vi "Set Margin.vi"(8 "error in (no error)":errorcluster, 9 "Margin":T1={"Type"=1, "Width"=40, "Sensitive"=TRUE, "Mask"=0, "Cursor"=2} {"Cursor" items=["Arrow"=2, "ReverseArrow"=7]; "Type" items=["Symbol", "Number", "BackColor", "ForeColor", "Text", "RightText", "Color"]}, 10 "Index":i32=1, 11 "ScintillaNET in":refnum<class "ScintillaNET.lvclass">) -> (0 "error out":errorcluster, 3 "ScintillaNET out":refnum<class "ScintillaNET.lvclass">)   [LabVIEW 2018, in "ScintillaNET.lvclass"]
uses:
  ScintillaNET.lvclass
  ScintillaNET.lvclass/ScintillaNET.ctl
  D:/project/hobby/LF2R/LabVIEW/source/ScintillaNET/dll/ScintillaNET.dll
  dll/ScintillaNET.dll
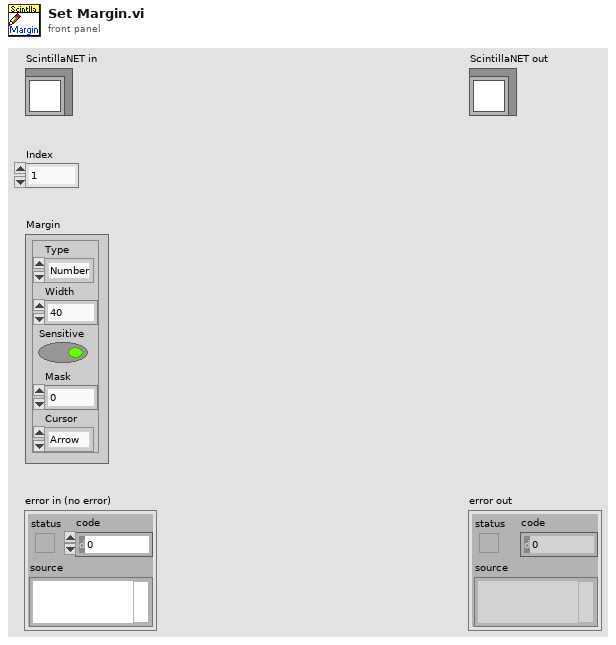
[diagram p1: front panel]
types:
  T1 = cluster{"Type":i32, "Width":i32, "Sensitive":bool, "Mask":u32, "Cursor":i32}
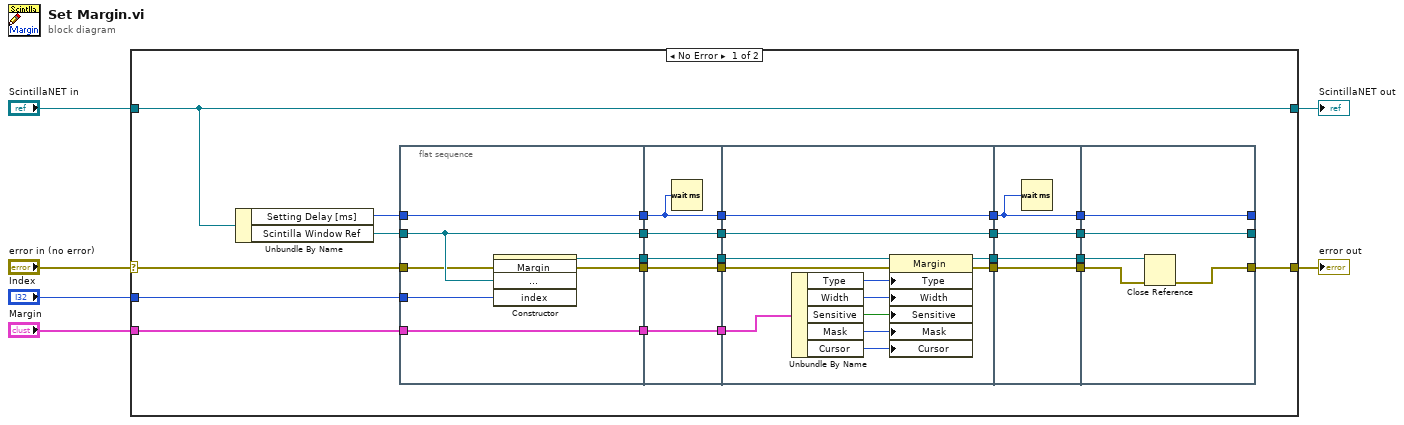
[diagram p0: block diagram]
diagram:
  n1 = case shown="No Error" "error in (no error)" {
    selector: "error in (no error)" -> [w8 w66]
    tunnel: [w7 w66] -> w5
    tunnel: [w15 w65] -> w3
    tunnel: "ScintillaNET in" -> [w15 w65]
    tunnel: "Margin" -> [w12 _]
    tunnel: "Index" -> [w11 _]
    frame No Error {
      n2 = Unbundle By Name(w15) -> ("Setting Delay [ms]"=w13:u32, "Scintilla Window Ref"=w14:refnum<k24>)
      n3 = flat-sequence {
        tunnel: w14 -> [w36]
        tunnel: [w38] -> w31
        tunnel: [w37] -> w30
        tunnel: [w36] -> w29
        tunnel: [w35] -> w28
        tunnel: w13 -> [w35]
        tunnel: w12 -> [w33]
        tunnel: w11 -> [w34]
        tunnel: [w33] -> w9
        tunnel: w8 -> [w32]
        tunnel: w31 -> [w43]
        tunnel: w30 -> [w42]
        tunnel: w29 -> [w41]
        tunnel: [w43] -> w27
        tunnel: [w42] -> w26
        tunnel: [w41] -> w25
        tunnel: w28 -> [w40]
        tunnel: [w40] -> w24
        tunnel: [w39] -> w10
        tunnel: w9 -> [w39]
        tunnel: w27 -> [w51]
        tunnel: w26 -> [w50]
        tunnel: w25 -> [w55]
        tunnel: w24 -> [w54]
        tunnel: [w52] -> w23
        tunnel: [w55] -> w22
        tunnel: [w54] -> w21
        tunnel: [w53] -> w20
        tunnel: w10 -> [w49]
        tunnel: w23 -> [w58]
        tunnel: w22 -> [w57]
        tunnel: w21 -> [w56]
        tunnel: w20 -> [w59]
        tunnel: [w59] -> w19
        tunnel: [w58] -> w18
        tunnel: [w57] -> w17
        tunnel: [w56] -> w16
        tunnel: [w63] -> _
        tunnel: [w64] -> _
        tunnel: w19 -> [w62]
        tunnel: w18 -> [w61]
        tunnel: w17 -> [w64]
        tunnel: w16 -> [w63]
        tunnel: [w60] -> w7
        frame #0 {
          n4 = constructor class="Margin"(error in=w32, "scintilla"=w36, "index"=w34) -> (reference out=w38:refnum<k24>, error out=w37:errorcluster)  [unwired: 2 in, 3 out]
        }
        frame #1 {
          n5 = Wait (ms)(milliseconds to wait=w40) -> ()  [unwired: 1 out]
        }
        frame #2 {
          n6 = Unbundle By Name(w49) -> ("Type"=w48:i32, "Width"=w47:i32, "Sensitive"=w46:bool, "Mask"=w45:u32, "Cursor"=w44:i32)
          n7 = property class="Margin"(reference=w51, error in=w50, "Type"=w48, "Width"=w47, "Sensitive"=w46, "Mask"=w45, "Cursor"=w44) -> (reference out=w53:refnum<k24>, error out=w52:errorcluster)
        }
        frame #3 {
          n8 = Wait (ms)(milliseconds to wait=w56) -> ()  [unwired: 1 out]
        }
        frame #4 {
          n9 = Close Reference(reference=w62, error in (no error)=w61) -> (error out=w60:errorcluster)
        }
      }
    }
    frame Error {
    }
  }
  "error out" <- w5
  "ScintillaNET out" <- w3
